vi "test2_guassian.vi"() -> ()   [LabVIEW 2018]
uses:
  <vilib>/imath/engines/lvmath2/RunTimeEngine/Managers/WorkSpace/UID Generator.vi
  <vilib>/imath/engines/lvmath2/RunTimeEngine/RunTimeType/NIMS_RunTimeType_From StrictType (excl LVString).vi
  <instcachedir>/0/NIMS_RunTimeType_From StrictType (excl LVString)_E7E34A65C99947108168652BAD14964D.lvgen/NIMS_RunTimeType_From StrictType (excl LVString)_E7E34A65C99947108168652BAD14964D_000.vi
  <vilib>/imath/engines/lvmath2/RunTimeEngine/LocalVariableDefStatement/MC_LocalVariableDefStatement_Display.vi
  <vilib>/imath/engines/lvmath2/RunTimeEngine/BuiltInFunctions/rand/NIMS_rand(I32,I32).vi
  <vilib>/imath/engines/lvmath2/RunTimeEngine/ArithmeticOperatorToken/NIMS_ArithmeticOperator_multmx(RV,M).vi
  <instcachedir>/0/NIMS_ArithmeticOperator_multmx(RV,M)_D6CB063A8E334F19B90764CB3E9B6C99.lvgen/NIMS_ArithmeticOperator_multmx(RV,M)_D6CB063A8E334F19B90764CB3E9B6C99_002.vi
  <vilib>/imath/engines/lvmath2/RunTimeEngine/ErrorHandling/NIMS_Error From Error Code.vi
  <vilib>/imathl/engines/lvmath/Functions/Error Handling/Create Error.vi
  <vilib>/imath/engines/lvmath/Functions/Error Handling/MergeErrorsWrapper.vi
  <vilib>/imath/engines/lvmath2/RunTimeSupport/NIMS_Complex To Real.vi
  <instcachedir>/0/NIMS_Complex To Real_DC07FF5F56D84FD694198341FF08C5E7.lvgen/NIMS_Complex To Real_DC07FF5F56D84FD694198341FF08C5E7_000.vi
  <vilib>/imath/engines/lvmath2/RunTimeSupport/NIMS_Get Any Vector_w Error - Matrix.vi
  <instcachedir>/0/NIMS_Get Any Vector_w Error - Matrix_1B26302039EC43C7B9FA287B1E12D88C.lvgen/NIMS_Get Any Vector_w Error - Matrix_1B26302039EC43C7B9FA287B1E12D88C_001.vi
  <vilib>/imath/engines/lvmath2/RunTimeEngine/BuiltInFunctions/density_kernel/NIMS_density_kernel(V,Var).vi
  <vilib>/imath/engines/lvmath2/RunTimeEngine/ErrorHandling/NIMS_Create Error From Enums.vi
  <vilib>/imath/engines/lvmath2/RunTimeEngine/BuiltInFunctions/histogram/NIMS_[M]=histogram(M).vi
  <vilib>/imath/engines/lvmath2/RunTimeEngine/IndexRead/NIMS M(S,$).vi
  <instcachedir>/0/NIMS M(S,$)_F24F360562DE41D8BE234322A2E15C65.lvgen/NIMS M(S,$)_F24F360562DE41D8BE234322A2E15C65_002.vi
  <instcachedir>/0/NIMS M(S,$)_F24F360562DE41D8BE234322A2E15C65.lvgen/NIMS M(S,$)_F24F360562DE41D8BE234322A2E15C65_000.vi
  <vilib>/imath/engines/lvmath2/RunTimeEngine/BuiltInFunctions/max/1 input/NIMS_max(CM).vi
  <instcachedir>/0/NIMS_max(CM)_7C352D5305924AD7A6AA4FE491F9CF6D.lvgen/NIMS_max(CM)_7C352D5305924AD7A6AA4FE491F9CF6D_000.vi
  <vilib>/imath/engines/lvmath2/RunTimeEngine/BuiltInFunctions/min/1 input/NIMS_min(CM).vi
  <instcachedir>/0/NIMS_min(CM)_1C1BDBC9E1754FFCB805E6CEF8E1CFA1.lvgen/NIMS_min(CM)_1C1BDBC9E1754FFCB805E6CEF8E1CFA1_000.vi
  <vilib>/imath/engines/lvmath2/RunTimeEngine/BuiltInFunctions/ones/NIMS_V=ones(I32,I32).vi
  <instcachedir>/0/NIMS_ArithmeticOperator_multmx(RV,M)_D6CB063A8E334F19B90764CB3E9B6C99.lvgen/NIMS_ArithmeticOperator_multmx(RV,M)_D6CB063A8E334F19B90764CB3E9B6C99_001.vi
  <vilib>/imath/engines/lvmath2/RunTimeEngine/IndexReplace/NIMS V(S)=M.vi
  <instcachedir>/0/NIMS V(S)=M_E1EF42F6623D44DBA15317938B9EE7AF.lvgen/NIMS V(S)=M_E1EF42F6623D44DBA15317938B9EE7AF_002.vi
  <vilib>/imath/engines/lvmath2/RunTimeEngine/ArithmeticOperatorToken/NIMS_ArithmeticOperator_times.vi
  <instcachedir>/0/NIMS_ArithmeticOperator_times_D7E4A7A4AD2C4409A0CE309D2741A5B4.lvgen/NIMS_ArithmeticOperator_times_D7E4A7A4AD2C4409A0CE309D2741A5B4_001.vi
  <vilib>/imath/engines/lvmath2/RunTimeEngine/BuiltInFunctions/mean/NIMS_CRow=mean(CM,I32).vi
  <vilib>/imath/engines/lvmath2/RunTimeEngine/IndexReplace/NIMS V(S)=V.vi
  <instcachedir>/0/NIMS V(S)=V_7FFD89C1C6FF454ABBE0B65E80594A53.lvgen/NIMS V(S)=V_7FFD89C1C6FF454ABBE0B65E80594A53_000.vi
  <vilib>/imath/engines/lvmath2/RunTimeEngine/BuiltInFunctions/std/NIMS_std(GM,RV).vi
  <instcachedir>/0/NIMS_std(GM,RV)_4F95049642544CB886F16E251B477F57.lvgen/NIMS_std(GM,RV)_4F95049642544CB886F16E251B477F57_000.vi
  <vilib>/imath/engines/lvmath2/RunTimeEngine/NodeEndStatement/NIMS_NodeEndStatement_Get Scalar.vi
  <instcachedir>/0/NIMS_NodeEndStatement_Get Scalar_89BDB89D2D624CD182477D809D857E40.lvgen/NIMS_NodeEndStatement_Get Scalar_89BDB89D2D624CD182477D809D857E40_000.vi
  <vilib>/imath/engines/lvmath2/RunTimeEngine/Managers/SymbolTable/Clear UID.vi
  <vilib>/imath/engines/lvmath2/RunTimeEngine/NodeEndStatement/NIMS_NodeEndStatement_Output.vi
  <instcachedir>/0/NIMS_NodeEndStatement_Output_53EC0D466D134D7ABD903AC30B43404B.lvgen/NIMS_NodeEndStatement_Output_53EC0D466D134D7ABD903AC30B43404B_010.vi
  <instcachedir>/0/NIMS_NodeEndStatement_Output_53EC0D466D134D7ABD903AC30B43404B.lvgen/NIMS_NodeEndStatement_Output_53EC0D466D134D7ABD903AC30B43404B_000.vi
  <instcachedir>/0/NIMS_NodeEndStatement_Output_53EC0D466D134D7ABD903AC30B43404B.lvgen/NIMS_NodeEndStatement_Output_53EC0D466D134D7ABD903AC30B43404B_005.vi
  <instcachedir>/0/NIMS_NodeEndStatement_Output_53EC0D466D134D7ABD903AC30B43404B.lvgen/NIMS_NodeEndStatement_Output_53EC0D466D134D7ABD903AC30B43404B_003.vi
  <vilib>/imath/engines/lvmath2/RunTimeEngine/ErrorHandling/NIMS_Finalize Error.vi
  <vilib>/imath/engines/lvmath2/RunTimeEngine/Managers/SymbolTable/NIMS_WorkSpace.lvlib
panel:
  out "point":dbl[][](graph)
  out "min":dbl
  out "max":dbl
  out "Compare":cluster{"t":dbl[], "y":dbl[]}[](graph)
  out "Err":dbl[](array[numeric])
  out "Ideal gaussian":cluster{"xi":dbl[], "f":dbl[]}(graph)
  out "line":dbl[][](graph)
  out "m":dbl[](array[numeric])
  in  "num":dbl=10000.0
  in  "a":dbl=4.0
  in  "mn":dbl=3.0
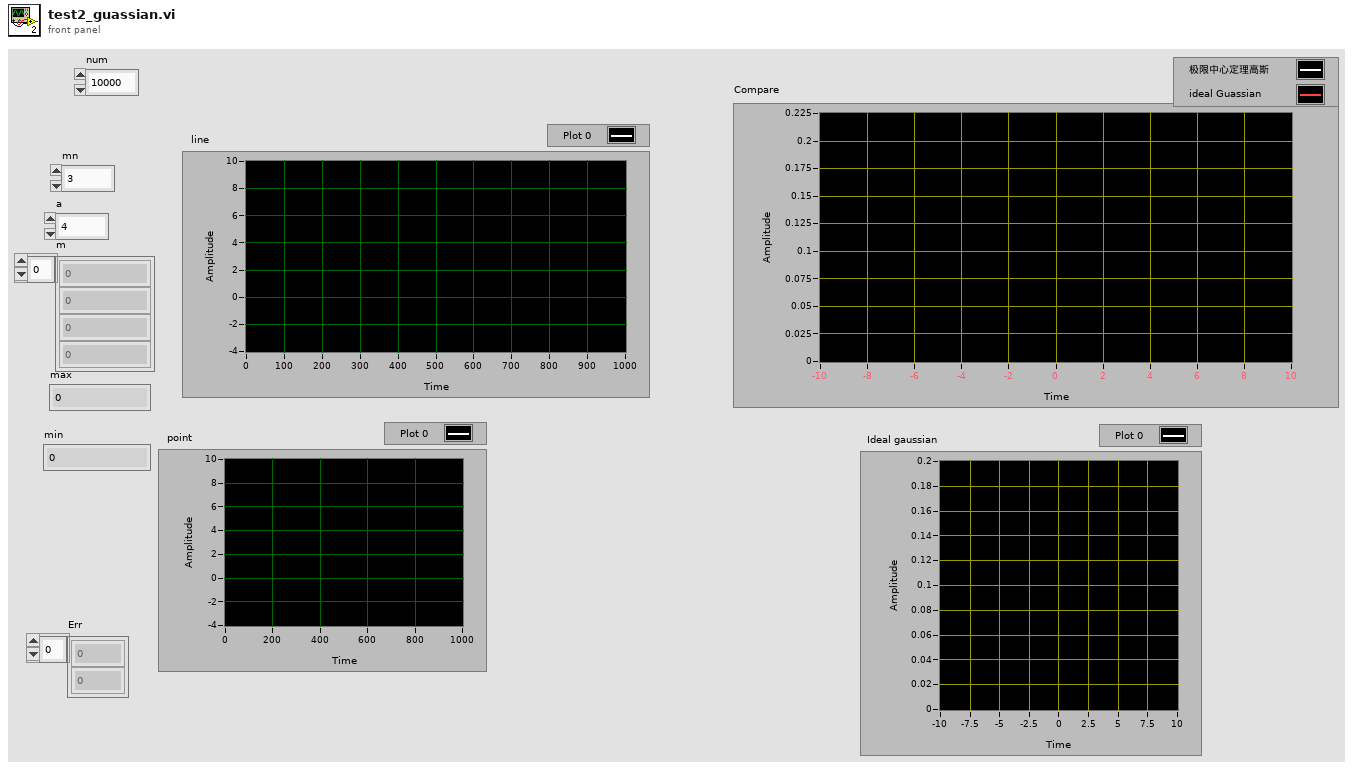
[diagram p1: front panel]
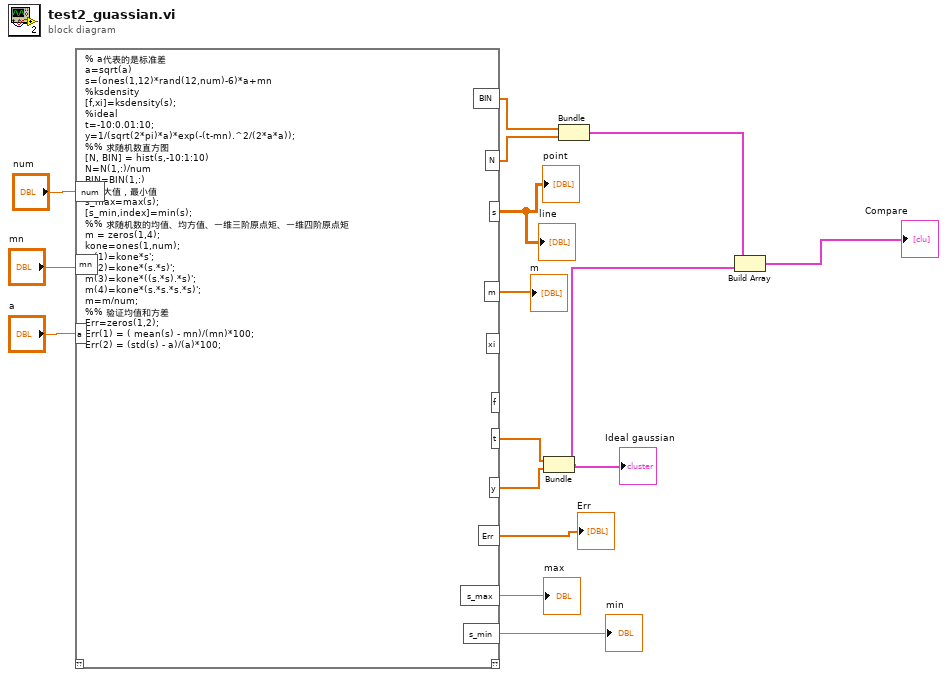
[diagram p0: block diagram]
diagram:
  n1 = mathscript code="% a代表的是标准差\na=sqrt(a)\ns=(ones(1,12)*rand(12,num)-6)*a+mn\n%ksdensity\n[f,xi]=ksdensity(s);\n%ideal\nt=-10:0.01:10;\ny=1/(sqrt(2*pi)*a)*exp(-(t-mn).^2/(2*a*a));\n%% 求随机数直方图\n[N, BIN] = hist(s,-10:1:10)\nN=N(1,:)/num\nBIN=BIN(1,:)\n%最大值，最小值\ns_max=max(s);\n[s_min,index]=min(s);\n%% 求随机数的均值、均方值、一维三阶原点矩、一维四阶原点矩\nm = zeros(1,4);        \nkone=ones(1,num);\nm(1)=kone*s';\nm(2)=kone*(s.*s)';\nm(3)=kone*((s.*s).*s)';\nm(4)=kone*(s.*s.*s.*s)';\nm=m/num;\n%% 验证均值和方差\nErr=zeros(1,2);\nErr(1) = ( mean(s) - mn)/(mn)*100;\nErr(2) = (std(s) - a)/(a)*100;"("num"="num", "mn"="mn", "a"="a") -> ("m"=→"m":cdb[], "s"=→"line" →"point":cdb[][], "N"=w7:dbl[], "BIN"=w8:dbl[], "t"=w10:dbl[], "y"=w11:cdb[], "Err"=→"Err":cdb[], "s_max"=→"max":sgl, "s_min"=→"min":sgl)  [unwired: 1 in, 3 out]
  n2 = Bundle("t"=w10, "y"=w11) -> (w5:cluster{"t":dbl[], "y":cdb[]})  [unwired: 1 in]
  "Ideal gaussian" <- w5
  n3 = Bundle("BIN"=w8, "N"=w7) -> (w1:cluster{"BIN":dbl[], "N":dbl[]})  [unwired: 1 in]
  n4 = Build Array(w1, w5) -> (→"Compare":cluster{"t":dbl[], "y":cdb[]}[])
